vi "timepulse.vi"(2 "de quantos segundos":i16=1) -> (1 "PULSO":bool)   [LabVIEW 2018]
panel:
  in  "Case Constant\n(See Context Help)":bool
  out "x+y":u32
  out "double precision float":dbl format="%#_10f"
  out "TIME ANTERIOR":u32
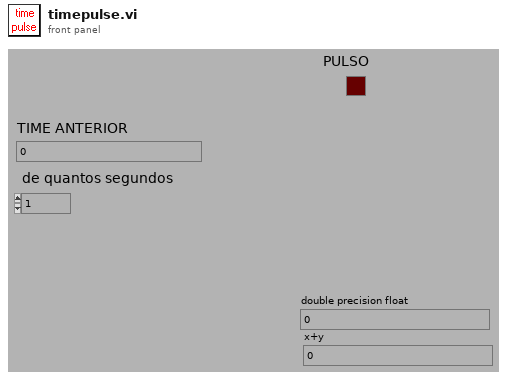
[diagram p1: front panel]
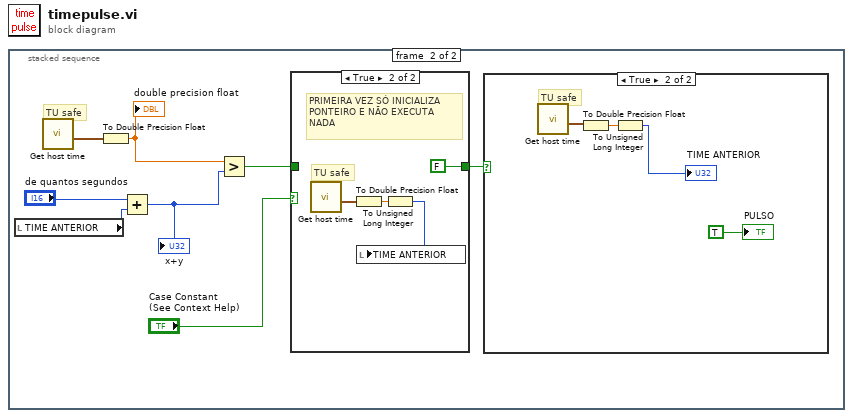
[diagram p0: block diagram]
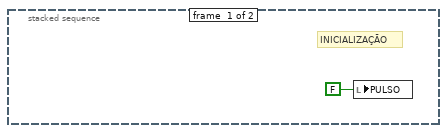
[diagram p2: hidden frame]
diagram:
  n1 = stacked-sequence {
    frame #0 {
      # "INICIALIZAÇÃO"
      n2 = local write "PULSO"(FALSE ("PULSO")) -> ()
    }
    frame #1 {
      # "TU safe"
      n3 = local read "TIME ANTERIOR"() -> (w6:u32)
      n4 = call "Get host time.vi"() -> ("BR current time"=w2:timestamp)  [unwired: 8 in, 3 out]
      n5 = To Double Precision Float(number=w2) -> (double precision float=w4:dbl)
      "double precision float" <- w4
      n6 = Add(x="de quantos segundos", y=w6) -> (x+y=w5:u32)
      "x+y" <- w5
      n7 = Greater?(x=w4, y=w5) -> (0:w9:bool)
      n8 = case shown="True" "Case Constant\n(See Context Help)" {
        tunnel: w9 -> [w10 _]
        tunnel: [w10 FALSE] -> w8
        frame False {
        }
        frame True {
          # "TU safe"
          # "PRIMEIRA VEZ SÓ INICIALIZA\nPONTEIRO E NÃO EXECUTA\nNADA"
          n9 = call "Get host time.vi"() -> ("BR current time"=w11:timestamp)  [unwired: 8 in, 3 out]
          n10 = To Double Precision Float(number=w11) -> (double precision float=w12:dbl)
          n11 = To Unsigned Long Integer(number=w12) -> (unsigned 32bit integer=w14:u32)
          n12 = local write "TIME ANTERIOR"(w14) -> ()
        }
      }
      n13 = case shown="True" w8 {
        frame False {
        }
        frame True {
          # "TU safe"
          n14 = call "Get host time.vi"() -> ("BR current time"=w15:timestamp)  [unwired: 8 in, 3 out]
          n15 = To Double Precision Float(number=w15) -> (double precision float=w16:dbl)
          n16 = To Unsigned Long Integer(number=w16) -> (unsigned 32bit integer=→"TIME ANTERIOR":u32)
          "PULSO" <- TRUE ("PULSO")
        }
      }
    }
  }
